vi "Set Headers.vi"(6 "Delimiter (,)":string=",", 7 "Buffer Header Size (5,000)":i32=5000, 8 "error in (no error)":errorcluster, 9 "Update Existing? (T)":bool=TRUE, 10 "Headers[]":string[](array[string]), 11 "File Path":path) -> (0 "error out":errorcluster, 3 "File Path dup":path)   [LabVIEW 2016, in "SLL Spreadsheet.lvlib" / "SLL CSV Logger.lvclass"]
doc: "Supports writing of 2D string with new line & comma to a spreadsheet file, which are not supported by LabVIEW's builtin function.\n\nIts functionality is similar to how Excel does it - it adds double quotes to cells which contains new line character, comma and double quotes. If the cell already has double quotes, it escapes it with one more double quotes."
uses:
  SLL CSV Logger.lvclass
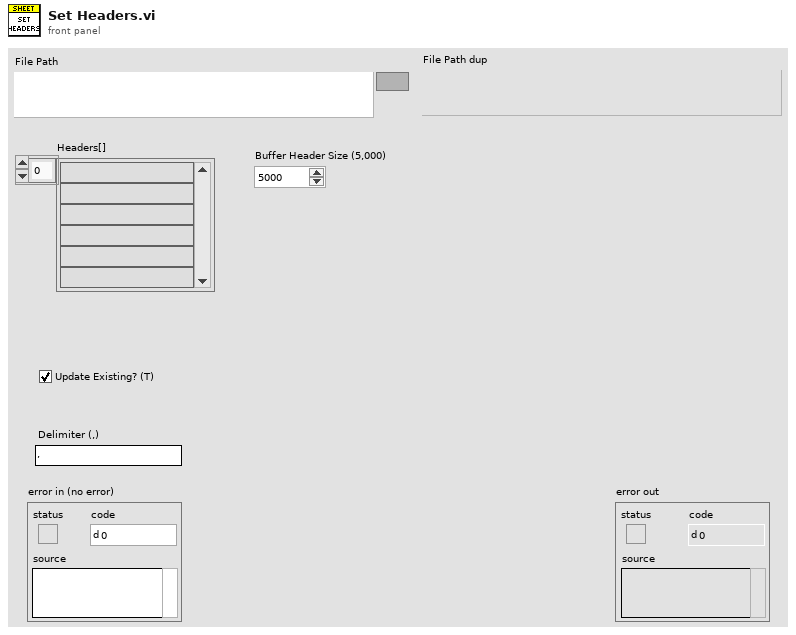
[diagram p1: front panel]
types:
  T1 = enum16{"open", "replace", "create", "open or create", "replace or create", "replace or create with confirmation"}
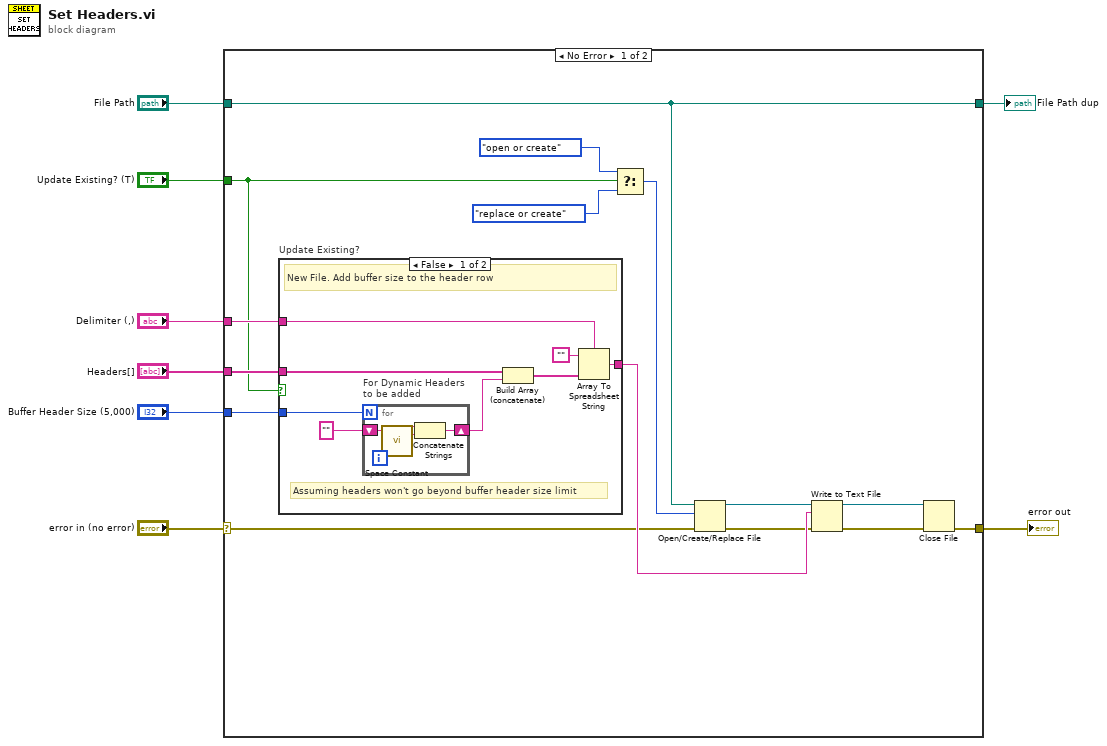
[diagram p0: block diagram]
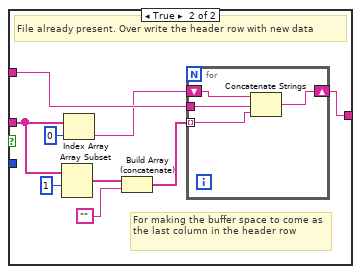
[diagram p2: hidden frame]
diagram:
  n1 = case shown="No Error" "error in (no error)" {
    selector: "error in (no error)" -> [w15 w49]
    tunnel: "Update Existing? (T)" -> [w10 _]
    tunnel: [w18 w49] -> w7
    tunnel: "Headers[]" -> [w11 _]
    tunnel: "Delimiter (,)" -> [w17 _]
    tunnel: "File Path" -> [w14 w48]
    tunnel: [w14 w48] -> w2
    tunnel: "Buffer Header Size (5,000)" -> [w9 _]
    frame No Error {
      n2 = case "Update Existing?" shown="False" w10 {
        tunnel: w17 -> [w31 w43]
        tunnel: [w30 w42] -> w16
        tunnel: w11 -> [w28 w39]
        tunnel: w9 -> [w24 _]
        frame False {
          # "Assuming headers won't go beyond buffer header size limit"
          # "New File. Add buffer size to the header row"
          n3 = for "For Dynamic Headers\nto be added" {
            N: w24 -> [_]
            shift-right: [w33] -> w26
            shift-left: "" -> [w32]
            n4 = call <vilib>:"Space Constant.vi"() -> ("String"=w34:string)
            n5 = Concatenate Strings(w32, w34) -> (w33:string)
          }
          n6 = Build Array (concatenate)(w28, w26) -> (w27:string[])
          n7 = Array To Spreadsheet String(delimiter (Tab)=w31, array=w27, 3:"") -> (spreadsheet string=w30:string)
        }
        frame True {
          # "For making the buffer space to come as the last column in the header row"
          # "File already present. Over write the header row with new data"
          n8 = Array Subset(array=w39, index=1) -> (w37:string[])  [unwired: 1 in]
          n9 = Index Array(array=w39, index=0) -> (element=w40:string)
          n10 = Build Array (concatenate)(w37, "") -> (w36:string[])
          n11 = for {
            tunnel: w36 -> [w46] mode=indexing
            tunnel: w43 -> [w47]
            shift-right: [w45] -> w42
            shift-left: w40 -> [w44]
            n12 = Concatenate Strings(w44, w47, w46) -> (w45:string)
          }
        }
      }
      n13 = Select ("function")(t=T1."open or create" ("operation (0:open)"), s=w10, f=T1."replace or create" ("operation (0:open)")) -> (s? t:f=w19:T1)
      n14 = Open/Create/Replace File(file path (use dialog)=w14, error in=w15, operation (0:open)=w19) -> (refnum out=w12:refnum<file>, error out=w13:errorcluster)  [unwired: 3 in, 1 out]
      n15 = Write to Text File(file (use dialog)=w12, text=w16, error in=w13) -> (refnum out=w21:refnum<file>, error out=w20:errorcluster)  [unwired: 1 in, 1 out]
      n16 = Close File(refnum=w21, error in=w20) -> (error out=w18:errorcluster)  [unwired: 1 out]
    }
    frame Error {
    }
  }
  "error out" <- w7
  "File Path dup" <- w2
